vi "Example Terminals 1.vi"() -> ()   [LabVIEW 2014]
panel:
  out "some number - control label":dbl
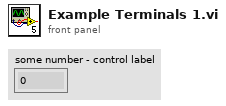
[diagram p1: front panel]
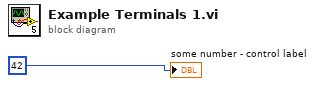
[diagram p0: block diagram]
diagram:
  "some number - control label" <- 42
